vi "Wave Manager.vi"(10 "Input Array":waveform(dbl)[](array[waveform]), 11 "data":waveform(dbl)) -> (2 "Waveform Graph Array":waveform(dbl)[](array[waveform]), 3 "Most Recent":dbl)   [LabVIEW 2016]
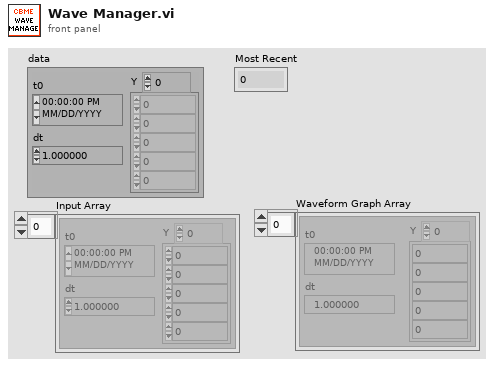
[diagram p1: front panel]
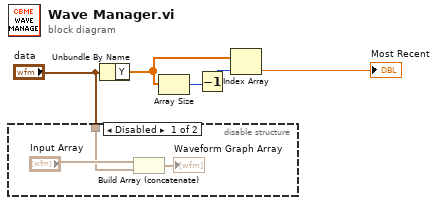
[diagram p0: block diagram]
diagram:
  n1 = disable-structure shown="Disabled" {
    disable-tunnel: "data" -> [w7 _]
    frame Disabled {
      n2 = Build Array (concatenate)("Input Array", w7) -> (→"Waveform Graph Array":waveform(dbl)[])
    }
    frame Enabled {
    }
  }
  n3 = Unbundle By Name("data") -> ("Y"=w4:dbl[])
  n4 = Array Size(array=w4) -> (size(s)=w2:i32)
  n5 = Decrement(x=w2) -> (x-1=w3:i32)
  n6 = Index Array(array=w4, index=w3) -> (element=→"Most Recent":dbl)
